vi "Reference_Test.vi"() -> (3 "Failed?":bool)   [LabVIEW 2017, in "WordManipulationTests.lvlib"]
uses:
  WordManipulationTests.lvlib
  Utilities/Parameters_Reference.ctl
  Utilities/WordManipulationLibrary.lvlib
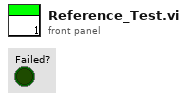
[diagram p1: front panel]
types:
  T1 = typedef "WordManipulationLibrary.lvlib/Parameters_Reference.ctl" = cluster{"Reference Move Mode":i32, "Start Search Forward":bool, "Stop on FWD Edge":bool, "Approach Forward":bool, "Velocity":dbl, "Acceleration":dbl}
  T2 = cluster{"Reference Move Mode":bool, "Start Search Forward":bool, "Stop on FWD Edge":bool, "Approach Forward":bool, "Velocity":bool, "Acceleration":bool}
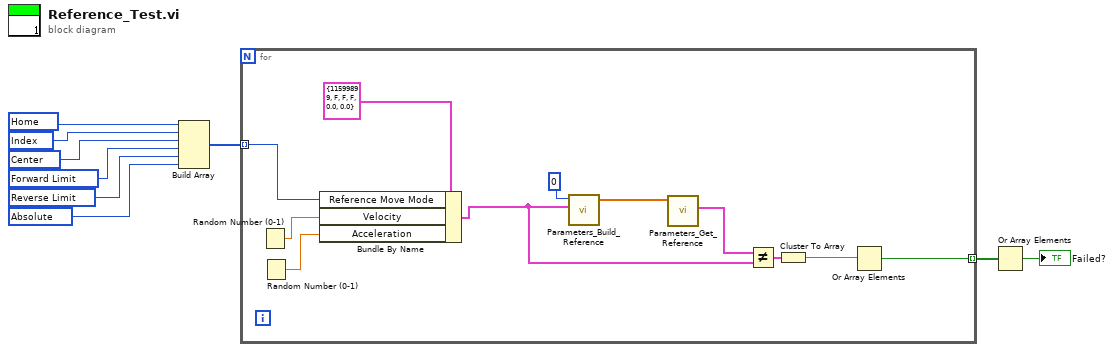
[diagram p0: block diagram]
diagram:
  w2 = 12648450 items=["Home"=11599899, "Index"=11599900, "Center"=11599901, "Forward Limit"=11599902, "Reverse Limit"=11599903, "Absolute"=12648450] ("Reference Move Mode")
  w3 = 11599903 items=["Home"=11599899, "Index"=11599900, "Center"=11599901, "Forward Limit"=11599902, "Reverse Limit"=11599903, "Absolute"=12648450] ("Reference Move Mode")
  w4 = 11599902 items=["Home"=11599899, "Index"=11599900, "Center"=11599901, "Forward Limit"=11599902, "Reverse Limit"=11599903, "Absolute"=12648450] ("Reference Move Mode")
  w5 = 11599901 items=["Home"=11599899, "Index"=11599900, "Center"=11599901, "Forward Limit"=11599902, "Reverse Limit"=11599903, "Absolute"=12648450] ("Reference Move Mode")
  w6 = 11599900 items=["Home"=11599899, "Index"=11599900, "Center"=11599901, "Forward Limit"=11599902, "Reverse Limit"=11599903, "Absolute"=12648450] ("Reference Move Mode")
  w7 = 11599899 items=["Home"=11599899, "Index"=11599900, "Center"=11599901, "Forward Limit"=11599902, "Reverse Limit"=11599903, "Absolute"=12648450] ("Reference Move Mode")
  n1 = Build Array(w7, w6, w5, w4, w3, w2) -> (w1:i32[])
  n2 = for {
    tunnel: [w17] -> w8 mode=indexing
    tunnel: w1 -> [w10] mode=indexing
    n3 = Random Number (0-1)() -> (number: 0 to 1=w19:dbl)
    n4 = Random Number (0-1)() -> (number: 0 to 1=w18:dbl)
    n5 = Bundle By Name(cluster=T1 {"Reference Move Mode"=11599899, "Start Search Forward"=FALSE, "Stop on FWD Edge"=FALSE, "Approach Forward"=FALSE, "Velocity"=0.0, "Acceleration"=0.0} ("Reference Move Parameters"), "Reference Move Mode"=w10, "Velocity"=w19, "Acceleration"=w18) -> (w13:T1)
    n6 = call "Parameters_Build_Reference.vi"("Reference Move Parameters"=w13, "Axis to command"=0) -> ("Parameters"=w11:dbl[])  [unwired: 9 in]
    n7 = call "Parameters_Get_Reference.vi"("Parameters"=w11) -> ("Reference Move Parameters"=w14:T1)  [unwired: 8 in, 2 out]
    n8 = Not Equal?(x=w14, y=w13) -> (x != y?=w15:T2)
    n9 = Cluster To Array(cluster=w15) -> (array=w12:bool[])
    n10 = Or Array Elements(Boolean array=w12) -> (logical OR=w17:bool)
  }
  n11 = Or Array Elements(Boolean array=w8) -> (logical OR=→"Failed?":bool)
